vi "CRYReport Flatten.vi"(11 "sData":string) -> (3 "flattened Data":string)   [LabVIEW 2013]
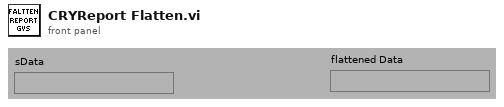
[diagram p1: front panel]
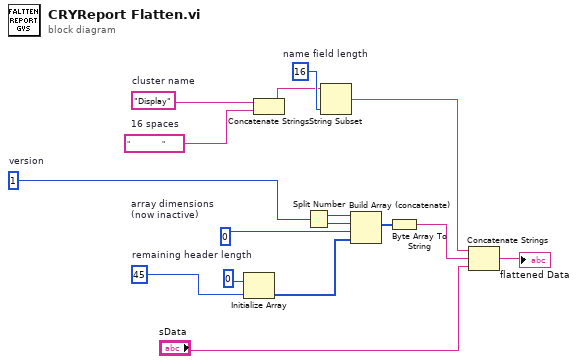
[diagram p0: block diagram]
diagram:
  w2 = u8 0  # array dimensions (now inactive)
  w5 = 16  # name field length
  w6 = "                "  # 16 spaces
  w7 = "Display"  # cluster name
  w12 = 45  # remaining header length
  w16 = u16 1  # version
  n1 = Initialize Array(u8 0, w12) -> (w8:u8[])
  n2 = Concatenate Strings(w7, w6) -> (w4:string)
  n3 = Split Number(x=w16) -> (hi(x)=w15:u8, lo(x)=w14:u8)
  n4 = String Subset(string=w4, length (rest)=w5) -> (substring=w3:string)  [unwired: 1 out]
  n5 = Build Array (concatenate)(w15, w14, w2, w8) -> (w11:u8[])
  n6 = Byte Array To String(unsigned byte array=w11) -> (string=w9:string)
  n7 = Concatenate Strings(w3, w9, "sData") -> (→"flattened Data":string)
